vi "sg Open Device.vi"(8 "error in (no error)":errorcluster, 11 "device":i32) -> (0 "error out":errorcluster, 2 "function return":u32(ring), 3 "device out":i32)   [LabVIEW 2014, in "VSG25A.lvlib"]
doc: "SG_API sgStatus sgOpenDevice(int *device);"
uses:
  VSG25A.lvlib
  sg_api.dll
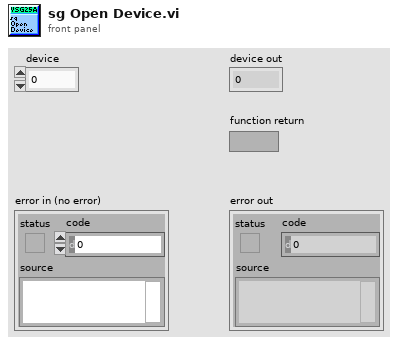
[diagram p1: front panel]
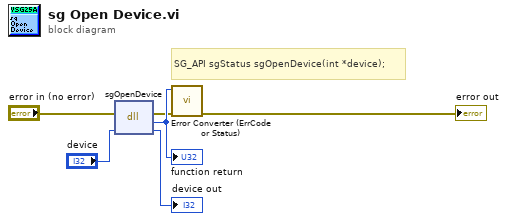
[diagram p0: block diagram]
diagram:
  # "SG_API sgStatus sgOpenDevice(int *device);"
  n1 = dll-call lib="C:/Users/M_LAPTOP/Desktop/Labview/practice/VSG25A/sg_lib/sg_api.*" fn="sgOpenDevice"(error in="error in (no error)", "device"="device") -> (error out=w2:errorcluster, w6:u32, "device"=→"device out":i32)  [unwired: 2 in, 1 out]
  "function return" <- w6
  n2 = call "Error Converter (ErrCode or Status).vi"("error in (no error)"=w2, "error code"=w6) -> ("error out"=→"error out":errorcluster)  [unwired: 9 in]
